vi "points_sub_frame.vi"(7 "Case select":string, 8 "felharmonikus N":i32=2, 9 "SNR window width [Hz]":dbl=0.4 format="%#_13g", 11 "path to binary file":path) -> (3 "output cluster":T1)   [LabVIEW 2019]
uses:
  <vilib>/regexp/Match Regular Expression.xnode
  <vilib>/Utility/file.llb/Read Delimited Spreadsheet (string).vi
panel:
  out "impulse szum/mean":cluster{"X":dbl, "Y":dbl}[](graph)
  out "Array":T2(array[cluster])
  out "header":T3
  out "impulse szum/time (bigger better)":cluster{"X":dbl, "Y":dbl}[](graph)
  out "X SNR 3":cluster{"X":dbl, "Y":dbl}[](graph)
  out "X SNR 4":cluster{"X":dbl, "Y":dbl}[](graph)
  out "X SNR":cluster{"X":dbl, "Y":dbl}[](graph)
  out "impulse mean":cluster{"X":dbl, "Y":dbl}[](graph)
  out "impulse sd":cluster{"X":dbl, "Y":dbl}[](graph)
  out "impulse szum":cluster{"X":dbl, "Y":dbl}[](graph)
  out "enable":bool
  out "end":timestamp
  out "start":timestamp
  out "state":string
  out "saved":string
  out "all rows":string[][](array[string])
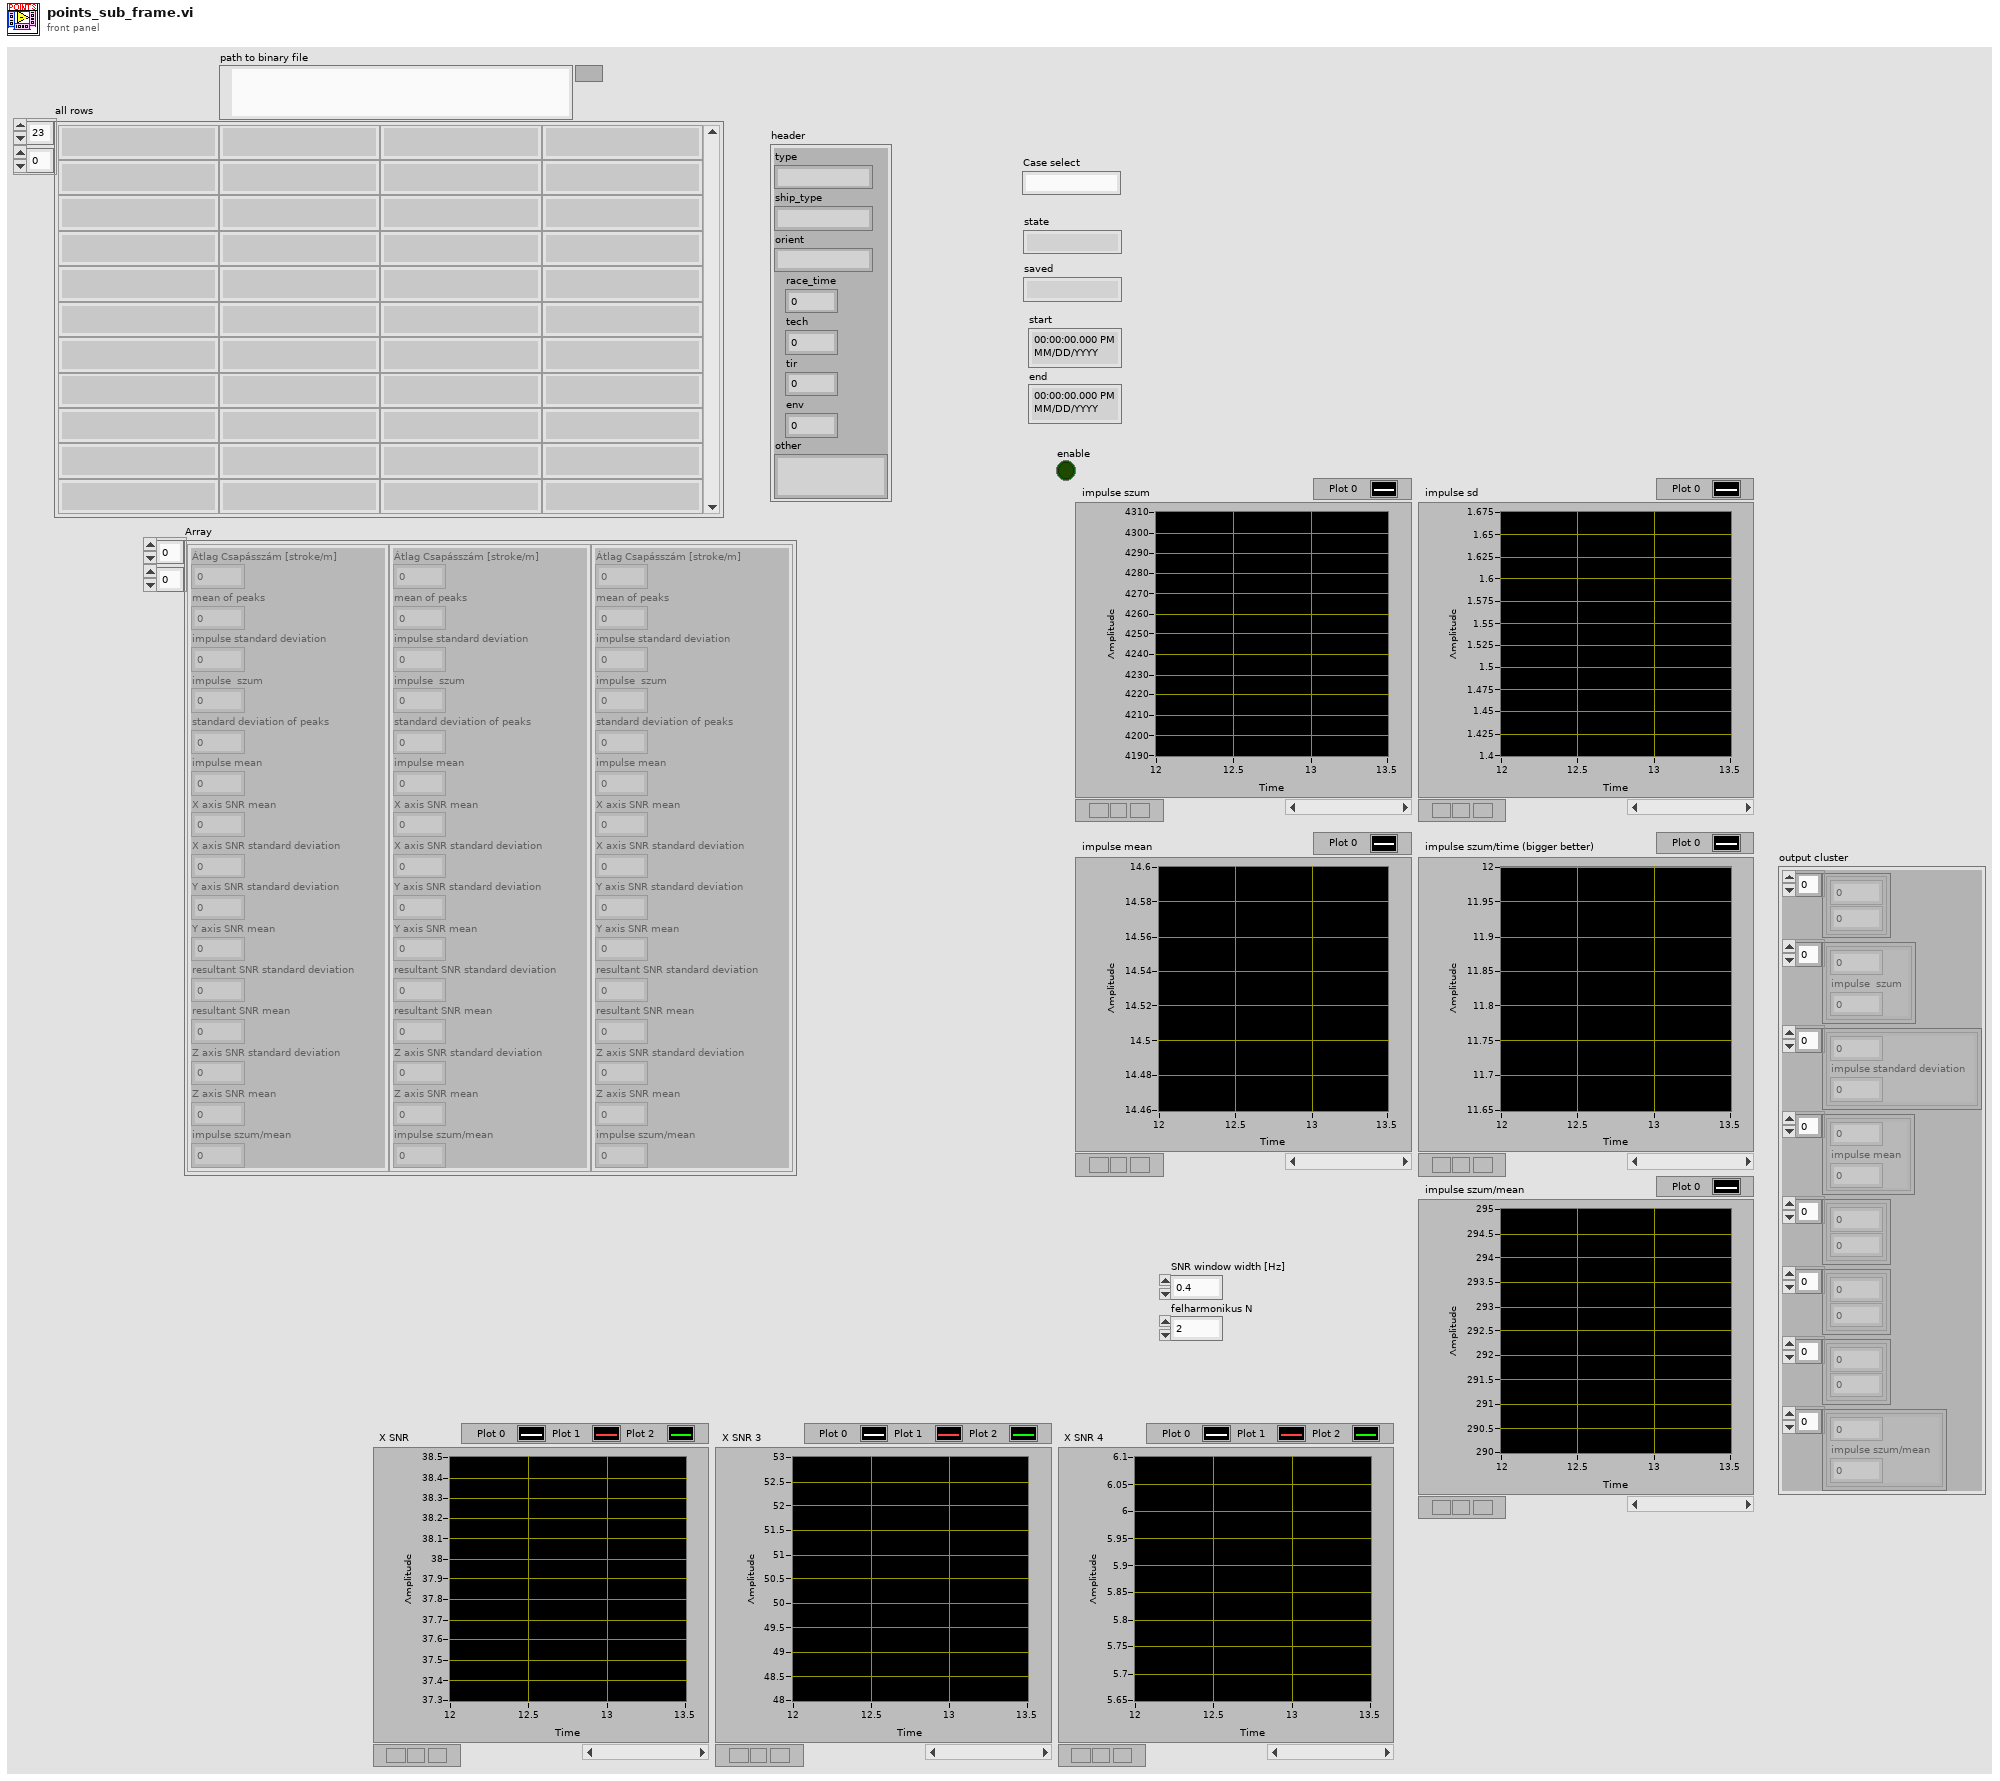
[diagram p1: front panel]
types:
  T1 = cluster{cluster{dbl, dbl}[], cluster{dbl, "impulse  szum":dbl}[], cluster{dbl, "impulse standard deviation":dbl}[], cluster{dbl, "impulse mean":dbl}[], cluster{dbl, dbl}[], cluster{dbl, dbl}[], cluster{dbl, dbl}[], cluster{dbl, "impulse szum/mean":dbl}[]}
  T2 = cluster{"Átlag Csapásszám [stroke/m]":dbl, "mean of peaks":dbl, "impulse standard deviation":dbl, "impulse  szum":dbl, "standard deviation of peaks":dbl, "impulse mean":dbl, "X axis SNR mean":dbl, "X axis SNR standard deviation":dbl, "Y axis SNR standard deviation":dbl, "Y axis SNR mean":dbl, "resultant SNR standard deviation":dbl, "resultant SNR mean":dbl, "Z axis SNR standard deviation":dbl, "Z axis SNR mean":dbl, "impulse szum/mean":dbl}[][]
  T3 = cluster{"type":string, "ship_type":string, "orient":string, "race_time":dbl, "tech":dbl, "tir":dbl, "env":dbl, "other":string}
  T4 = cluster{cluster{dbl, "impulse szum/time":dbl}[], cluster{dbl, "impulse  szum":dbl}[], cluster{dbl, "impulse standard deviation":dbl}[], cluster{dbl, "impulse mean":dbl}[], cluster{dbl, dbl}[], cluster{dbl, dbl}[], cluster{dbl, dbl}[]}
  T5 = typedef "control_time_informations.ctl" = cluster{"starting time":timestamp, "ending time":timestamp, "dt[s]":dbl, "sampling rate [Hz]":dbl, "length":dbl}
  T6 = typedef "control_all_in_one_package.ctl" = cluster{"memory structure":T7, "actigraph settings":T8, "time informations":T5, "measurement data":T9}
  T7 = typedef "control_memory_structure.ctl" = cluster{"length of metadata [byte]":i32, "length of page [byte]":i32, "length of measurement data on page [byte]":i32, "length of dataset [byte]":i32}
  T8 = typedef "control_measurement_settings.ctl" = cluster{"sampling frequency [Hz]":dbl, "measurement interval [± g]":i32, "high precision?":bool, "number of pages":i32, "rate code":i32, "range code":i32, "id":i32}
  T9 = typedef "control_measurement_data.ctl" = cluster{"number of samples per axis":i32, "timestamp array":dbl[], "offset array":dbl[], "x, y, z axis data":waveform(dbl)[], "normalised magnitude of acceleartion vectors":waveform(dbl), "calibration coefficients":T10, "statistics":T11, "battery voltage":waveform(dbl), "magnitude of acceleartion vectors":waveform(dbl)}
  T10 = typedef "control_calibration_coefficients.ctl" = cluster{"Sx":dbl, "Ox":dbl, "Sy":dbl, "Oy":dbl, "Sz":dbl, "Oz":dbl}
  T11 = typedef "control_statistics.ctl" = cluster{"mean of x axis acceleration":dbl, "standard devation of x axis acceleration":dbl, "mean of y axis acceleration":dbl, "standard devation of y axis acceleration":dbl, "mean of z axis acceleration":dbl, "standard devation of z axis acceleration":dbl, "mean of normalised magnitude of acceleration":dbl, "standard devation of normalised magnitude of acceleration":dbl}
  T12 = cluster{"path to binary file":path, "Start Cursor":timestamp, "Sec":dbl, "crossing level":dbl, "threshold":dbl, "avg window size":i32, "peak detect width":i32, "invert":bool, "SNR window width [Hz]":dbl, "felharmonikus N":i32, "End cursor":timestamp}
  T13 = cluster{"Átlag Csapásszám [stroke/m]":dbl, "mean of peaks":dbl, "impulse standard deviation":dbl, "impulse  szum":dbl, "standard deviation of peaks":dbl, "impulse mean":dbl, "X axis SNR mean":dbl, "X axis SNR standard deviation":dbl, "Y axis SNR standard deviation":dbl, "Y axis SNR mean":dbl, "resultant SNR standard deviation":dbl, "resultant SNR mean":dbl, "Z axis SNR standard deviation":dbl, "Z axis SNR mean":dbl, "impulse szum/mean":dbl}
  T14 = cluster{"Átlag Csapásszám [stroke/m]":dbl, "mean of peaks":dbl, "impulse standard deviation":dbl, "impulse  szum":dbl, "standard deviation of peaks":dbl, "impulse mean":dbl, "X axis SNR mean":dbl, "X axis SNR standard deviation":dbl, "Y axis SNR standard deviation":dbl, "Y axis SNR mean":dbl, "resultant SNR standard deviation":dbl, "resultant SNR mean":dbl, "Z axis SNR standard deviation":dbl, "Z axis SNR mean":dbl, "impulse szum/mean":dbl}[]
  T15 = cluster{"tech":dbl, "impulse standard deviation":dbl}
  T16 = cluster{cluster{"tech":dbl, dbl}[], cluster{"tech":dbl, "impulse  szum":dbl}[], cluster{"tech":dbl, "impulse standard deviation":dbl}[], cluster{"tech":dbl, "impulse mean":dbl}[], cluster{dbl, "SNR":dbl}[], cluster{dbl, "SNR":dbl}[], cluster{dbl, "SNR":dbl}[], cluster{"tech":dbl, "impulse szum/mean":dbl}[]}
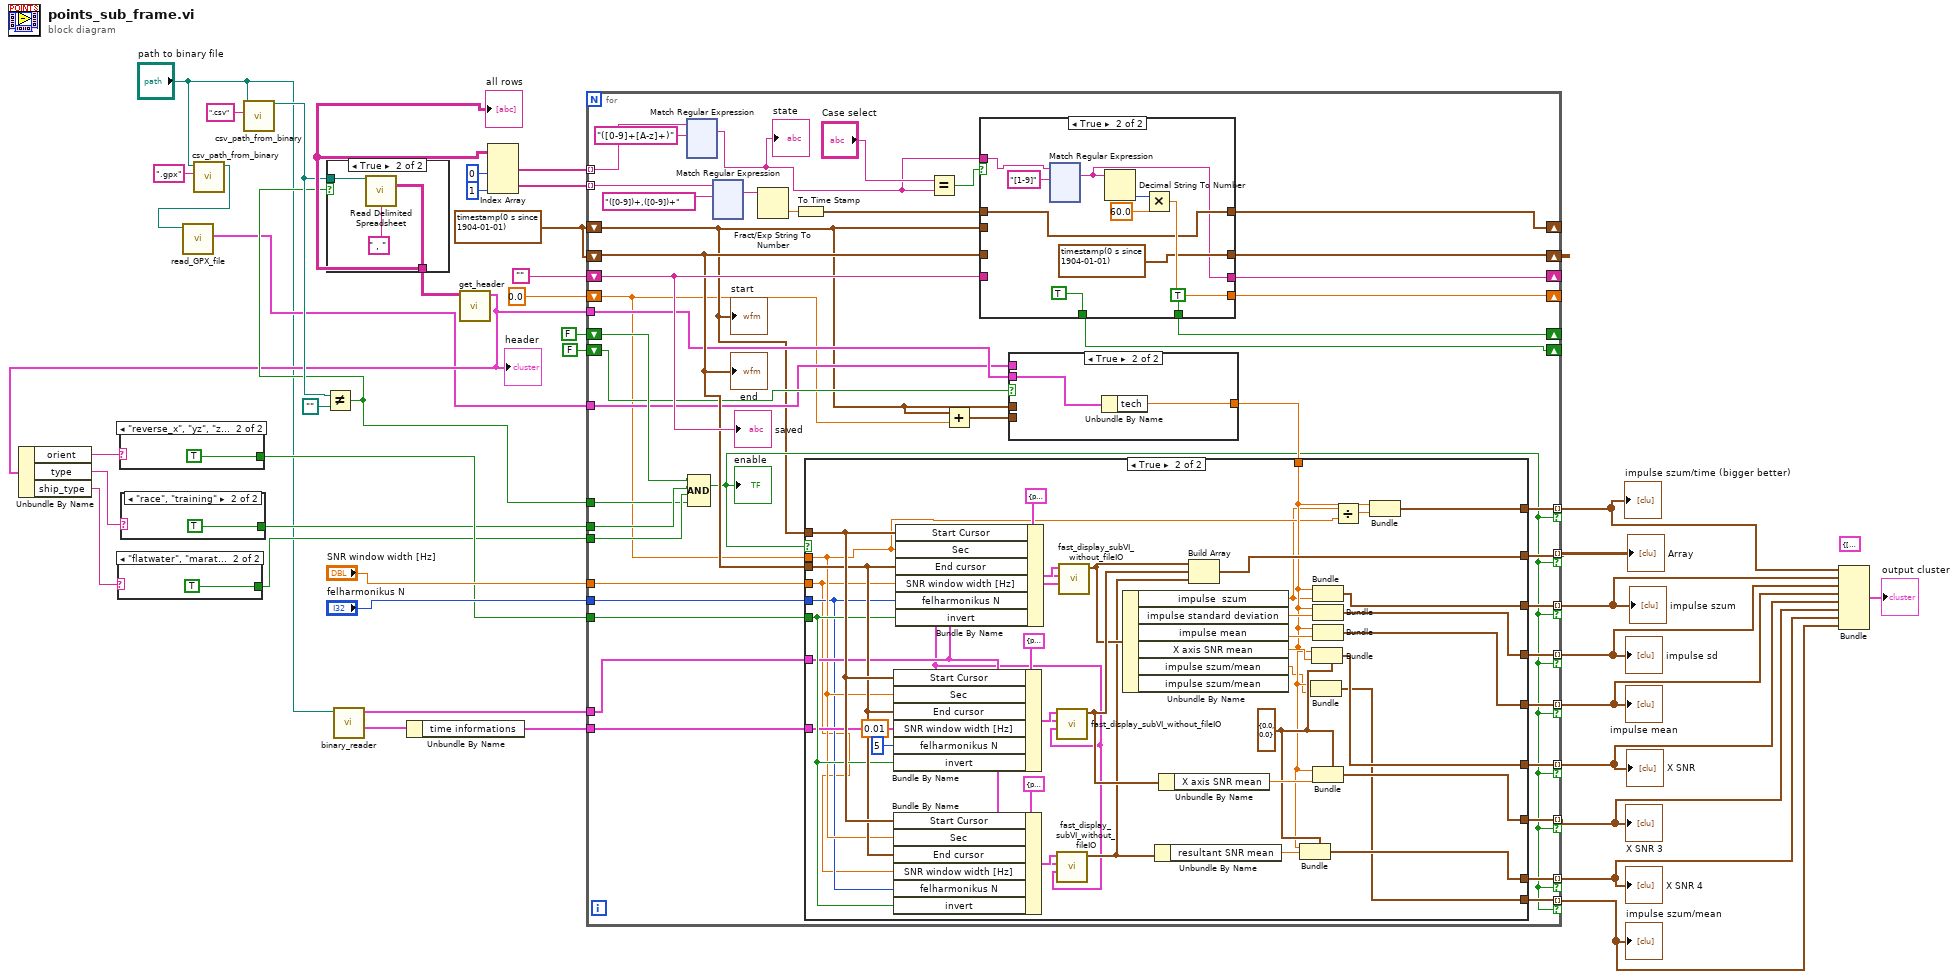
[diagram p0: block diagram]
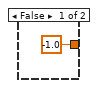
[diagram p2: hidden frame]
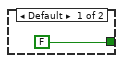
[diagram p6: hidden frame]
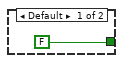
[diagram p7: hidden frame]
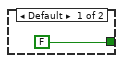
[diagram p8: hidden frame]
diagram:
  w13 = timestamp(0 s since 1904-01-01)
  (unwired) T4 {[], [], [], [], [], [], []} ("output cluster")
  n1 = call "csv_path_from_binary.vi"("extension"=".gpx", "path to binary file"="path to binary file") -> ("path to spec. ext."=w10:path)  [unwired: 9 in]
  n2 = call "read_GPX_file.vi"("GPX File Path"=w10) -> ("lat/lon position"=w9:cluster{timestamp[], dbl[], dbl[]})  [unwired: 3 in, 3 out]
  n3 = call "csv_path_from_binary.vi"("extension"=".csv", "path to binary file"="path to binary file") -> ("path to spec. ext."=w17:path)  [unwired: 9 in]
  n4 = Not Equal?(x=w17, y=path "") -> (x != y?=w16:bool)
  n5 = case shown="True" w16 {
    tunnel: [_ w42] -> w18
    tunnel: w17 -> [_ w41]
    frame False {
    }
    frame True {
      n6 = call-poly <vilib>:"Read Delimited Spreadsheet.vi"("file path (dialog if empty)"=w41, "delimiter (\\t)"=" , " ("delimiter (\\t)")) -> ("all rows"=w42:string[][])  [unwired: 8 in, 5 out]
    }
  }
  "all rows" <- w18
  n7 = call "binary_reader.vi"("path to binary file"="path to binary file") -> ("time informations"=w3:T5, "all in one package"=w4:T6)  [unwired: 7 in, 1 out]
  n8 = Unbundle By Name(w3) -> ("time informations"=w2:T5)
  n9 = call "get_header.vi"("all rows"=w18) -> ("header"=w14:T3)  [unwired: 10 in]
  "header" <- w14
  n10 = Unbundle By Name(w14) -> ("orient"=w32:string, "type"=w23:string, "ship_type"=w21:string)
  n11 = case shown="\"flatwater\", \"marathon\"" w21 {
    tunnel: [FALSE TRUE] -> w20
    frame Default {
    }
    frame "flatwater", "marathon" {
    }
  }
  n12 = case shown="\"reverse_x\", \"yz\", \"z\"" w32 {
    tunnel: [FALSE TRUE] -> w31
    frame Default {
    }
    frame "reverse_x", "yz", "z" {
    }
  }
  n13 = case shown="\"race\", \"training\"" w23 {
    tunnel: [FALSE TRUE] -> w22
    frame Default {
    }
    frame "race", "training" {
    }
  }
  n14 = Index Array(array=w18, index (col) #1=0 ("disabled index (col)"), index (col) #2=1 ("index (col)")) -> (element #1=w39:string[], element #2=w40:string[])  [unwired: 2 in]
  n15 = for {
    tunnel: w40 -> [w90] mode=indexing
    tunnel: w39 -> [w85] mode=indexing
    shift-right: [w88] -> _
    shift-left: w13 -> [w54]
    shift-right: [w87] -> _
    shift-left: w13 -> [w78]
    shift-right: [w86] -> _
    shift-left: "" -> [w83]
    shift-right: [w65] -> _
    shift-left: 0.0 ("Sec") -> [w53]
    shift-right: [w82] -> _
    shift-left: FALSE -> [w69]
    tunnel: "SNR window width [Hz]" -> [w81]
    tunnel: "felharmonikus N" -> [w80]
    tunnel: w31 -> [w79]
    tunnel: [w77] -> w8 mode=indexing if=w55
    tunnel: [w76] -> w29 mode=indexing if=w55
    tunnel: [w75] -> w28 mode=indexing if=w55
    tunnel: [w74] -> w27 mode=indexing if=w55
    tunnel: [w73] -> w26 mode=indexing if=w55
    tunnel: [w72] -> w25 mode=indexing if=w55
    tunnel: [w71] -> w24 mode=indexing if=w55
    tunnel: [w70] -> w30 mode=indexing if=w55
    tunnel: w22 -> [w68]
    tunnel: w20 -> [w67]
    tunnel: w16 -> [w66]
    tunnel: w14 -> [w64]
    shift-right: [w62] -> _
    shift-left: FALSE -> [w61]
    tunnel: w9 -> [w57]
    tunnel: [w56] -> w7 mode=indexing if=w55
    tunnel: w4 -> [w51]
    tunnel: w2 -> [w50]
    n16 = xnode "Match Regular Expression"("input string"=w85, "regular expression"="([0-9]+[A-z]+)") -> ("whole match"=w59:string)  [unwired: 4 in, 4 out]
    "state" <- w59
    n17 = Compound Arithmetic op=AND(w69, w68, w67, w66) -> (w55:bool)
    "enable" <- w55
    n18 = xnode "Match Regular Expression"("input string"=w90, "regular expression"="([0-9])+,([0-9])+") -> ("whole match"=w92:string)  [unwired: 4 in, 4 out]
    n19 = Fract/Exp String To Number(string=w92) -> (number=w91:dbl)  [unwired: 3 in, 1 out]
    n20 = To Time Stamp(1:w91) -> (0:w89:timestamp)
    n21 = Equal?(x="Case select", y=w59) -> (x = y?=w58:bool)
    n22 = Add(x=w54, y=w53) -> (x+y=w52:timestamp)
    n23 = case shown="True" w58 {
      tunnel: [w249 w257] -> w88
      tunnel: w89 -> [_ w257]
      tunnel: [w250 timestamp(0 s since 1904-01-01) ("f")] -> w87
      tunnel: [w251 w253] -> w86
      tunnel: w83 -> [w251 _]
      tunnel: [_ w258] -> w65
      tunnel: w78 -> [w250 _]
      tunnel: w54 -> [w249 _]
      tunnel: [_ TRUE] -> w82
      tunnel: [_ TRUE] -> w62
      tunnel: w59 -> [_ w252]
      frame False {
      }
      frame True {
        n24 = xnode "Match Regular Expression"("input string"=w252, "regular expression"="[1-9]") -> ("whole match"=w253:string)  [unwired: 4 in, 4 out]
        n25 = Decimal String To Number(string=w253) -> (number=w259:i32)  [unwired: 2 in, 1 out]
        n26 = Multiply(x=w259, y=60.0) -> (x*y=w258:dbl)
      }
    }
    n27 = case shown="True" w61 {
      tunnel: w54 -> [_ _]
      tunnel: w52 -> [_ _]
      tunnel: [-1.0 ("tech") w95] -> w63
      tunnel: w64 -> [_ w96]
      tunnel: w57 -> [_ _]
      frame False {
      }
      frame True {
        n28 = Unbundle By Name(w96) -> ("tech"=w95:dbl)
      }
    }
    n29 = case shown="True" w55 {
      tunnel: w54 -> [_ w128]
      tunnel: w78 -> [_ w127]
      tunnel: w53 -> [_ w103]
      tunnel: w81 -> [_ w99]
      tunnel: w80 -> [_ w100]
      tunnel: w79 -> [_ w126]
      tunnel: w63 -> [_ w108]
      tunnel: [_ w121] -> w77
      tunnel: [_ w120] -> w76
      tunnel: [_ w119] -> w75
      tunnel: [_ w118] -> w74
      tunnel: [_ w113] -> w73
      tunnel: [_ w112] -> w72
      tunnel: [_ w111] -> w71
      tunnel: [_ w109] -> w70
      tunnel: [_ w106] -> w56
      tunnel: w51 -> [_ w105]
      tunnel: w50 -> [_ w104]
      frame False {
      }
      frame True {
        w110 = cluster{dbl, "SNR":dbl} {0.0, "SNR"=0.0} ("cluster")
        n30 = Bundle By Name(cluster=T12 {"path to binary file"=path "C:/Users/Lenovo/Desktop/szakdoga/data", "Start Cursor"=timestamp(0 s since 1904-01-01), "Sec"=60.0, "crossing level"=0.0, "threshold"=0.35, "avg window size"=5, "peak detect width"=30, "invert"=FALSE, "SNR window width [Hz]"=0.5, "felharmonikus N"=2, "End cursor"=timestamp(0 s since 1904-01-01)} ("input cluster"), "Start Cursor"=w128, "Sec"=w103, "End cursor"=w127, "SNR window width [Hz]"=0.01, "felharmonikus N"=5, "invert"=w126) -> (w131:T12)
        n31 = Bundle By Name(cluster=T12 {"path to binary file"=path "C:/Users/Lenovo/Desktop/szakdoga/data", "Start Cursor"=timestamp(0 s since 1904-01-01), "Sec"=60.0, "crossing level"=0.0, "threshold"=0.35, "avg window size"=5, "peak detect width"=30, "invert"=FALSE, "SNR window width [Hz]"=0.5, "felharmonikus N"=2, "End cursor"=timestamp(0 s since 1904-01-01)} ("input cluster"), "Start Cursor"=w128, "Sec"=w103, "End cursor"=w127, "SNR window width [Hz]"=w99, "felharmonikus N"=w100, "invert"=w126) -> (w130:T12)
        n32 = Bundle By Name(cluster=T12 {"path to binary file"=path "C:/Users/Lenovo/Desktop/szakdoga/data", "Start Cursor"=timestamp(0 s since 1904-01-01), "Sec"=60.0, "crossing level"=0.0, "threshold"=0.35, "avg window size"=5, "peak detect width"=30, "invert"=FALSE, "SNR window width [Hz]"=0.5, "felharmonikus N"=2, "End cursor"=timestamp(0 s since 1904-01-01)} ("input cluster"), "Start Cursor"=w128, "Sec"=w103, "End cursor"=w127, "SNR window width [Hz]"=w99, "felharmonikus N"=w100, "invert"=w126) -> (w134:T12)
        n33 = call "fast_display_subVI_without_fileIO.vi"("time informations"=w104, "acc waveform array"=w105, "input cluster"=w131) -> ("data cluster"=w123:T13)  [unwired: 8 in]
        n34 = call "fast_display_subVI_without_fileIO.vi"("time informations"=w104, "acc waveform array"=w105, "input cluster"=w130) -> ("data cluster"=w114:T13)  [unwired: 8 in]
        n35 = call "fast_display_subVI_without_fileIO.vi"("time informations"=w104, "acc waveform array"=w105, "input cluster"=w134) -> ("data cluster"=w122:T13)  [unwired: 8 in]
        n36 = Unbundle By Name(w122) -> ("impulse  szum"=w102:dbl, "impulse standard deviation"=w124:dbl, "impulse mean"=w125:dbl, "X axis SNR mean"=w117:dbl, "impulse szum/mean"=w107:dbl)  [unwired: 1 out]
        n37 = Unbundle By Name(w114) -> ("resultant SNR mean"=w115:dbl)
        n38 = Unbundle By Name(w123) -> ("X axis SNR mean"=w116:dbl)
        n39 = Build Array(w122, w123, w114) -> (w121:T14)
        n40 = Bundle(cluster=w110, w108, "SNR"=w115) -> (w111:cluster{dbl, "SNR":dbl})
        n41 = Bundle("tech"=w108, "impulse szum/mean"=w107) -> (w106:cluster{"tech":dbl, "impulse szum/mean":dbl})  [unwired: 1 in]
        n42 = Bundle(cluster=w110, w108, "SNR"=w117) -> (w113:cluster{dbl, "SNR":dbl})
        n43 = Bundle("tech"=w108, "impulse  szum"=w102) -> (w120:cluster{"tech":dbl, "impulse  szum":dbl})  [unwired: 1 in]
        n44 = Bundle("tech"=w108, "impulse standard deviation"=w124) -> (w119:T15)  [unwired: 1 in]
        n45 = Bundle("tech"=w108, "impulse mean"=w125) -> (w118:cluster{"tech":dbl, "impulse mean":dbl})  [unwired: 1 in]
        n46 = Bundle(cluster=w110, w108, "SNR"=w116) -> (w112:cluster{dbl, "SNR":dbl})
        n47 = Divide(x=w102, y=w103) -> (x/y=w101:dbl)
        n48 = Bundle("tech"=w108, w101) -> (w109:cluster{"tech":dbl, dbl})  [unwired: 1 in]
      }
    }
    "saved" <- w83
    "start" <- w54
    "end" <- w78
  }
  "impulse szum" <- w29
  "impulse sd" <- w28
  "impulse mean" <- w27
  "X SNR" <- w26
  "X SNR 4" <- w24
  "X SNR 3" <- w25
  "impulse szum/time (bigger better)" <- w30
  "Array" <- w8
  "impulse szum/mean" <- w7
  n49 = Bundle(w30, w29, w28, w27, w26, w25, w24, w7) -> (→"output cluster":T16)  [unwired: 1 in]
